vi "Close Apps.vi"(1 "error in":errorcluster) -> (0 "error out":errorcluster)   [LabVIEW 2012, in "Design Server.lvlib"]
uses:
  Design Server.lvlib
  AutoCAD cmds.ctl
  Word cmd.ctl
  Mathcad15 cmds.ctl
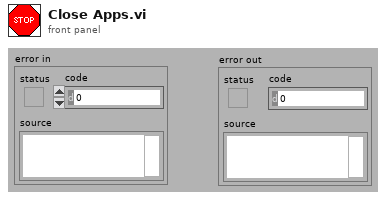
[diagram p1: front panel]
types:
  T1 = typedef "Design Server.lvlib/Mathcad15 cmds.ctl" = enum16{"Open Mathcad", "Execute Method", "Quit Mathcad"}
  T2 = typedef "Design Server.lvlib/Word cmd.ctl" = enum16{"Initialize", "Create Reports", "Quit"}
  T3 = typedef "Design Server.lvlib/AutoCAD cmds.ctl" = enum16{"Open AutoCAD", "Create Drawing", "Quit"}
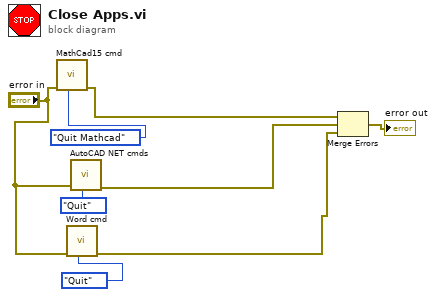
[diagram p0: block diagram]
diagram:
  n1 = call "MathCad15 cmd.vi"("Mathcad15 cmds"=Mathcad15_cmds."Quit Mathcad", "error in"="error in") -> ("first error out"=w4:errorcluster)  [unwired: 7 in, 2 out]
  n2 = call "Word cmd.vi"("Word cmd"=Word_cmd."Quit", "Error In (no error)"="error in") -> ("error out"=w2:errorcluster)  [unwired: 8 in, 1 out]
  n3 = call "AutoCAD NET cmds.vi"("AutoCAD cmd"=AutoCAD_cmds."Quit", "error in (no error)"="error in") -> ("error out"=w3:errorcluster)  [unwired: 8 in, 1 out]
  n4 = Merge Errors(w4, w3, w2) -> (→"error out":errorcluster)
